vi "Config Camera Settings.vi"   [LabVIEW 2014]
uses:
  <vilib>/Rock Robotics/WPI/Camera/WPI_CameraExposure Values.ctl
  Robot Global Data.vi
types:
  T1 = typedef "Dashboard Control Data.ctl" = cluster{"Cam Exposure":dbl}
  T2 = typedef "WPI_CameraDevRef.ctl" = cluster{"Camera Address":string, "CameraStatus":errorcluster}
  T3 = typedef "WPI_CameraExposure Values.ctl" = enum16{"Auto", "Flicker-free 50 Hz", "Flicker-free 60 Hz", "Hold current", "Custom"}
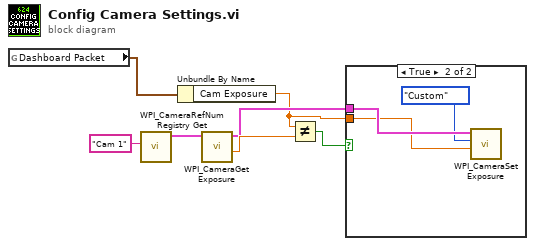
[diagram p0: block diagram]
diagram:
  n1 = global read "Robot Global Data.vi" "Dashboard Packet"() -> (w5:T1)
  n2 = call <vilib>:"WPI_CameraRefNum Registry Get.vi"("refnum name"="Cam 1") -> ("CameraDevRef"=w6:T2)  [unwired: 9 in, 1 out]
  n3 = Unbundle By Name(w5) -> ("Cam Exposure"=w1:dbl)
  n4 = call <vilib>:"WPI_CameraGet Exposure.vi"("CameraDevRef"=w6) -> ("Exposure (%)"=w4:dbl, "CameraDevRef Out"=w2:T2)  [unwired: 7 in, 2 out]
  n5 = Not Equal?(x=w1, y=w4) -> (x != y?=w3:bool)
  n6 = case shown="True" w3 {
    tunnel: w2 -> [_ w10]
    tunnel: w1 -> [_ w9]
    frame False {
    }
    frame True {
      n7 = call <vilib>:"WPI_CameraSet Exposure.vi"("Exposure (%)"=w9, "Exposure"=WPI_CameraExposure_Values."Custom", "CameraDevRef"=w10) -> ()  [unwired: 7 in, 2 out]
    }
  }
